vi "stop.vi"(8 "error in (no error)":errorcluster, 10 "stop":bool, 11 "CameraNetworkController in":refnum<class "CameraNetworkController.lvclass">) -> (0 "error out":errorcluster, 2 "stopped?":bool, 3 "CameraNetworkController out":refnum<class "CameraNetworkController.lvclass">)   [LabVIEW 2011, in "Hardware.lvlib" / "HWControllers.lvlib" / "CameraNetworkController.lvclass"]
uses:
  CameraNetworkController.lvclass
  NetworkClient/NetworkServer.lvclass
panel:
  out "element":string
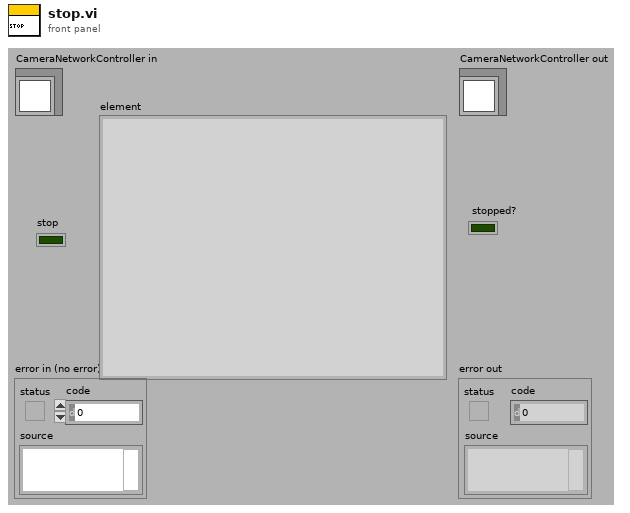
[diagram p1: front panel]
types:
  T1 = cluster{"Message":enum16{"Idle", "initialise", "configureAcquisition", "setTemperature", "getTemperature", "start", "stop", "sendImage", "close", "error", "ExitApp", "getAcquisitionStatus"}, "Data":variant}
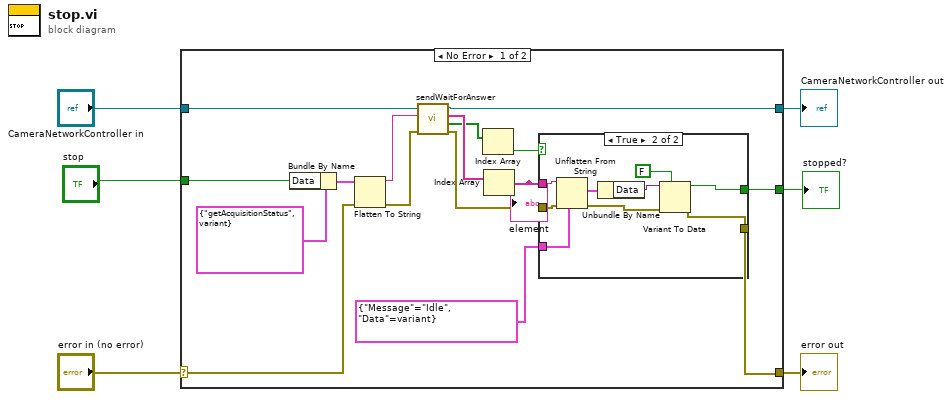
[diagram p0: block diagram]
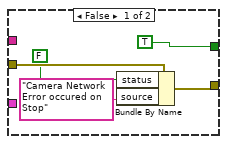
[diagram p2: hidden frame]
diagram:
  n1 = case shown="No Error" "error in (no error)" {
    selector: "error in (no error)" -> [w19 w38]
    tunnel: [w14 w38] -> w5
    tunnel: [w16 w37] -> w3
    tunnel: "CameraNetworkController in" -> [w22 w37]
    tunnel: "stop" -> [w7 _]
    tunnel: [w15 _] -> w1
    frame No Error {
      n2 = Bundle By Name(cluster=T1 {"Message"=enum."getAcquisitionStatus", "Data"=variant}, "Data"=w7) -> (w21:T1)
      n3 = Flatten To String(anything=w21, error in (no error)=w19) -> (data string=w20:string, error out=w12:errorcluster)  [unwired: 3 out]
      n4 = call "sendWaitForAnswer.vi"("error in (no error)"=w12, "message"=w20, "NetworkServer in"=w22) -> ("error out"=w13:errorcluster, "valid?"=w10:bool[], "answers"=w17:string[], "NetworkServer out"=w16:refnum<class "CameraNetworkController.lvclass">)  [unwired: 5 in]
      n5 = Index Array(array=w10) -> (element=w11:bool)  [unwired: 1 in]
      n6 = Index Array(array=w17) -> (element=w18:string)  [unwired: 1 in]
      "element" <- w18
      n7 = case shown="True" w11 {
        tunnel: T1 {"Message"=enum."Idle", "Data"=variant} -> [_ w36]
        tunnel: w18 -> [_ w35]
        tunnel: [TRUE w31] -> w15
        tunnel: [w24 w30] -> w14
        tunnel: w13 -> [w26 w28]
        frame False {
          n8 = Bundle By Name(cluster=w26, "status"=FALSE, "source"="Camera Network Error occured on Stop") -> (w24:errorcluster)
        }
        frame True {
          n9 = Unflatten From String(type=w36, binary string=w35, error in (no error)=w28) -> (value=w34:T1, error out=w29:errorcluster)  [unwired: 2 in, 1 out]
          n10 = Unbundle By Name(w34) -> ("Data"=w33:variant)
          n11 = Variant To Data(error in=w29, type=FALSE, Variant=w33) -> (data=w31:bool, error out=w30:errorcluster)
        }
      }
    }
    frame Error {
    }
  }
  "error out" <- w5
  "CameraNetworkController out" <- w3
  "stopped?" <- w1
